vi "Get Channel Configuration.vi"(8 "error in (no error)":errorcluster, 11 "Channel Item Ref in":T4 format="%.0x") -> (0 "error out":errorcluster, 2 "Channel Configuration":T1={"Channel#"=0, "Measurement Type"=0, "Position_LVDT_Properties"={"Minimum Value"=-0.1, "Maximum Value"=0.1, "Excitation Source"=10200, "Excitation Wire Mode"=4, "Excitation Frequency"=2500.0, "Excitation Value"=1.0, "Units"=10219, "Sensitivity"=50.0, "Sensitivity Units"=12506, "Excitation Sense"=16095}, "Position_RVDT_Properties"={"Minimum Value"=-70.0, "Maximum Value"=70.0, "Excitation Source"=10200, "Excitation Wire Mode"=4, "Excitation Frequency"=2500.0, "Excitation Value"=1.0, "Units"=10146, "Sensitivity"=50.0, "Sensitivity Units"=12507, "Excitation Sense"=16095}} {"Position_RVDT_Properties"."Sensitivity Units" items=["mVolts/Volt/Degree"=12507, "mVolts/Volt/Radian"=12508]; "Position_RVDT_Properties"."Units" items=["Degrees"=10146, "Radians"=10273, "From Custom Scale"=10065]; "Position_RVDT_Properties"."Excitation Sense" items=["Local"=16095, "Remote"=16096]; "Position_RVDT_Properties"."Excitation Source" items=["Internal"=10200, "External"=10167, "None"=10230]; "Position_RVDT_Properties"."Excitation Wire Mode" items=["4-Wire"=4, "5-Wire"=5, "6-Wire"=6]; "Position_LVDT_Properties"."Excitation Sense" items=["Local"=16095, "Remote"=16096]; "Position_LVDT_Properties"."Excitation Source" items=["Internal"=10200, "External"=10167, "None"=10230]; "Position_LVDT_Properties"."Excitation Wire Mode" items=["4-Wire"=4, "5-Wire"=5, "6-Wire"=6]; "Position_LVDT_Properties"."Units" items=["Meters"=10219, "Inches"=10379, "From Custom Scale"=10065]; "Position_LVDT_Properties"."Sensitivity Units" items=["mVolts/Volt/mMeter"=12506, "mVolts/Volt/0.001 Inch"=12505]; "Measurement Type" items=["Position LVDT", "Position RVDT"]}, 3 "Channel Item Ref out":T4 format="%.0x")   [LabVIEW 2020, in "NI PXIe-4340 Shared.lvlib"]
uses:
  NI PXIe-4340 Shared.lvlib
  <vilib>/NI VeriStand/Custom Device API/Custom Device Item Ref.ctl
  Channel Configuration.ctl
  Position_LVDT_Properties.ctl
  Position_RVDT_Properties.ctl
  Constants.vi
  <vilib>/NI VeriStand/Custom Device API/Get Item Property (Variant).vi
  <vilib>/NI VeriStand/Custom Device API/Get Item Property (I32).vi
  <vilib>/NI VeriStand/Custom Device API/Custom Device API.lvlib
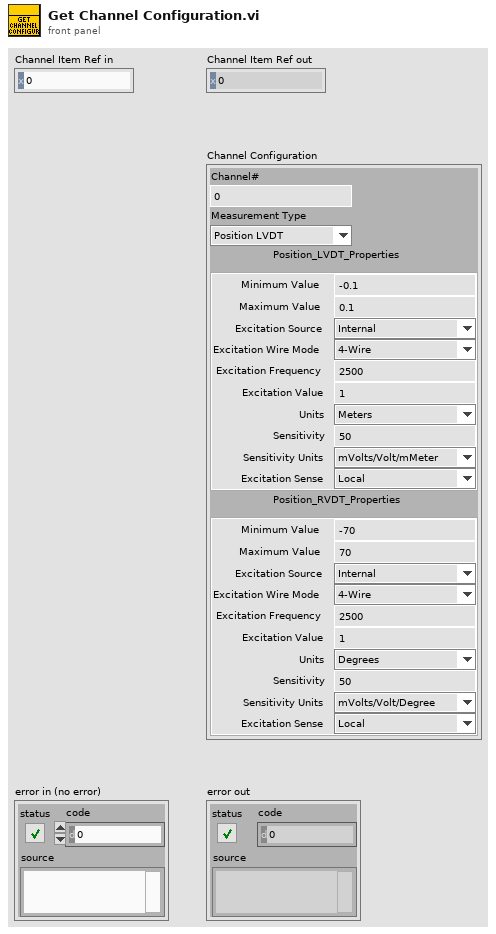
[diagram p1: front panel]
types:
  T1 = typedef "NI PXIe-4340 Shared.lvlib/Channel Configuration.ctl" = cluster{"Channel#":i32, "Measurement Type":i32, "Position_LVDT_Properties":T2, "Position_RVDT_Properties":T3}
  T2 = typedef "NI PXIe-4340 Shared.lvlib/Position_LVDT_Properties.ctl" = cluster{"Minimum Value":dbl, "Maximum Value":dbl, "Excitation Source":i32, "Excitation Wire Mode":i32, "Excitation Frequency":dbl, "Excitation Value":dbl, "Units":i32, "Sensitivity":dbl, "Sensitivity Units":i32, "Excitation Sense":i32}
  T3 = typedef "NI PXIe-4340 Shared.lvlib/Position_RVDT_Properties.ctl" = cluster{"Minimum Value":dbl, "Maximum Value":dbl, "Excitation Source":i32, "Excitation Wire Mode":i32, "Excitation Frequency":dbl, "Excitation Value":dbl, "Units":i32, "Sensitivity":dbl, "Sensitivity Units":i32, "Excitation Sense":i32}
  T4 = typedef "Custom Device API.lvlib/Custom Device Item Ref.ctl" = u64
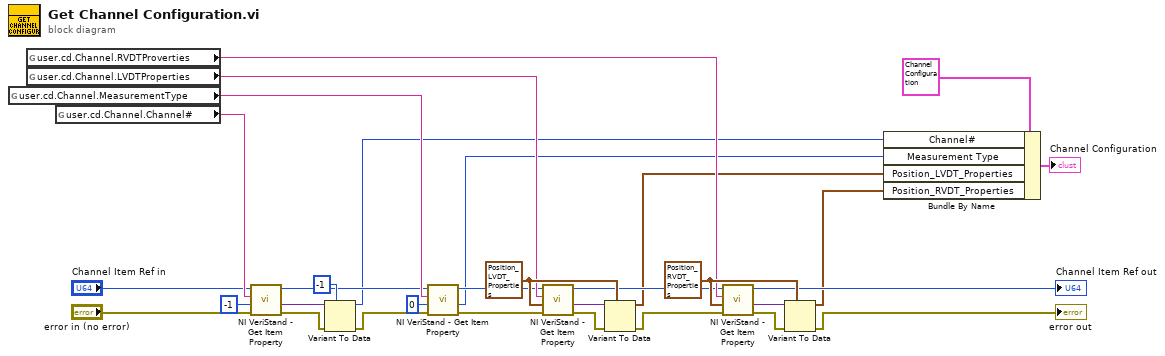
[diagram p0: block diagram]
diagram:
  w31 = T3 {"Minimum Value"=-70.0, "Maximum Value"=70.0, "Excitation Source"=10200, "Excitation Wire Mode"=4, "Excitation Frequency"=2500.0, "Excitation Value"=1.0, "Units"=10146, "Sensitivity"=50.0, "Sensitivity Units"=12507, "Excitation Sense"=16095} ("Position_RVDT_Properties")
  w19 = T2 {"Minimum Value"=-0.1, "Maximum Value"=0.1, "Excitation Source"=10200, "Excitation Wire Mode"=4, "Excitation Frequency"=2500.0, "Excitation Value"=1.0, "Units"=10219, "Sensitivity"=50.0, "Sensitivity Units"=12506, "Excitation Sense"=16095} ("Position_LVDT_Properties")
  n1 = global read "Constants.vi" "user.cd.Channel.MeasurementType"() -> (w9:string)
  n2 = global read "Constants.vi" "user.cd.Channel.RVDTProverties"() -> (w15:string)
  n3 = global read "Constants.vi" "user.cd.Channel.LVDTProperties"() -> (w13:string)
  n4 = global read "Constants.vi" "user.cd.Channel.Channel#"() -> (w25:string)
  n5 = call-poly <vilib>:"NI VeriStand - Get Item Property.vi"("error in (no error)"="error in (no error)", "Default Value"=-1, "Property Name"=w25, "Item Ref in"="Channel Item Ref in") -> ("error out"=w28:errorcluster, "Value"=w27:variant, "Item Ref out"=w7:T4)  [unwired: 4 in, 1 out]
  n6 = Variant To Data(error in=w28, type=-1, Variant=w27) -> (data=w5:i32, error out=w6:errorcluster)
  n7 = call-poly <vilib>:"NI VeriStand - Get Item Property.vi"("error in (no error)"=w6, "Default Value"=0, "Property Name"=w9, "Item Ref in"=w7) -> ("error out"=w12:errorcluster, "Value"=w4:i32, "Item Ref out"=w11:T4)  [unwired: 4 in, 1 out]
  n8 = call-poly <vilib>:"NI VeriStand - Get Item Property.vi"("error in (no error)"=w12, "Default Value"=w19, "Property Name"=w13, "Item Ref in"=w11) -> ("error out"=w17:errorcluster, "Value"=w18:variant, "Item Ref out"=w14:T4)  [unwired: 4 in, 1 out]
  n9 = Variant To Data(error in=w17, type=w19, Variant=w18) -> (data=w3:T2, error out=w16:errorcluster)
  n10 = call-poly <vilib>:"NI VeriStand - Get Item Property.vi"("error in (no error)"=w16, "Default Value"=w31, "Property Name"=w15, "Item Ref in"=w14) -> ("error out"=w20:errorcluster, "Value"=w21:variant, "Item Ref out"=→"Channel Item Ref out":T4)  [unwired: 4 in, 1 out]
  n11 = Variant To Data(error in=w20, type=w31, Variant=w21) -> (data=w2:T3, error out=→"error out":errorcluster)
  n12 = Bundle By Name(cluster=T1 {"Channel#"=0, "Measurement Type"=0, "Position_LVDT_Properties"={"Minimum Value"=-0.1, "Maximum Value"=0.1, "Excitation Source"=10200, "Excitation Wire Mode"=4, "Excitation Frequency"=2500.0, "Excitation Value"=1.0, "Units"=10219, "Sensitivity"=50.0, "Sensitivity Units"=12506, "Excitation Sense"=16095}, "Position_RVDT_Properties"={"Minimum Value"=-70.0, "Maximum Value"=70.0, "Excitation Source"=10200, "Excitation Wire Mode"=4, "Excitation Frequency"=2500.0, "Excitation Value"=1.0, "Units"=10146, "Sensitivity"=50.0, "Sensitivity Units"=12507, "Excitation Sense"=16095}} ("Channel Configuration"), "Channel#"=w5, "Measurement Type"=w4, "Position_LVDT_Properties"=w3, "Position_RVDT_Properties"=w2) -> (→"Channel Configuration":T1)
